vi "MM9.ProcCases.vi"(0 "i ref in":refnum<vi>, 1 "selector":string, 2 "Data":T1, 3 "call cluster":T3={"Object"="", "Selector"="", "CallType"=enum."synchronous", "Async Object"="", "Async Selector"="", "Data Descriptor"="", "Data"=[], "Error #"=0, "Expire"=0}, 5 "error in (no error)":errorcluster) -> (14 "i ref out":refnum<vi>, 17 "answer cluster":T3={"Object"="", "Selector"="", "CallType"=enum."synchronous", "Async Object"="", "Async Selector"="", "Data Descriptor"="", "Data"=[], "Error #"=0, "Expire"=0}, 19 "error out":errorcluster)   [LabVIEW 2014, in "MM9.lvlib"]
doc: "This method is called by a process from within the default case in the event loop. The methods of a class that are linked to events will be called from THIS method. Add your code here."
uses:
  MM9.lvlib
  CS_Core/CSSystem/CoreDefs/CoreDefs.call_type.ctl
  CS_Core/BaseProcess/BaseProcess.descriptor string definition.ctl
  CS_Core/CSSystem/CoreDefs/CoreDefs.rawDataType.ctl
  MM9.status.ctl
  CS_Core/CSSystem/CoreLib/CoreLib.byte array 2 string.vi
  CS_Core/CSSystem/CoreLib/CoreLib.string 2 byte array.vi
  CS_Core/BaseProcess/BaseProcess.lvlib
  CS_Core/CSSystem/CoreLib/CoreLib.lvlib
  CS_Core/CSSystem/CSSystemLib/CSSystemLib.lvlib
  CSlibraries-extern/DimLVEvent/LVDimInterface/LVDimInterface.lvlib
panel:
  in  "MMStatus":T2=enum."config"
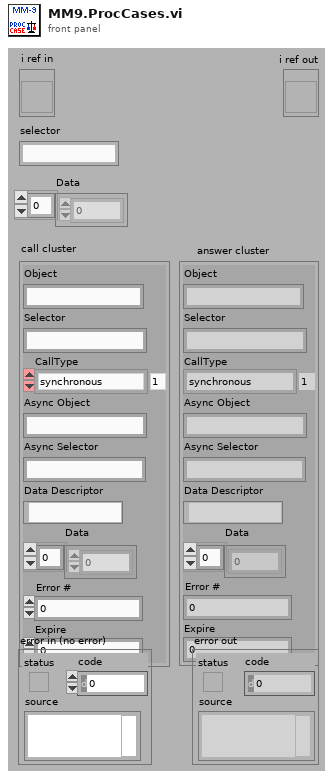
[diagram p1: front panel]
types:
  T1 = typedef "CoreDefs.rawDataType.ctl" = i8[]
  T2 = typedef "MM9.lvlib/MM9.status.ctl" = enum16{"loaded", "load_error", "config", "config_error", "init", "init_error", "data_reset", "data_reset_error", "running", "start_error", "run_error", "abort_requested", "aborted", "stop_requested", "stopped", "stop_error", "Connected", "NOTConnected"}
  T3 = typedef "CoreDefs.call_type.ctl" = cluster{"Object":string, "Selector":string, "CallType":enum16{"simple", "synchronous", "asynchronous"}, "Async Object":string, "Async Selector":string, "Data Descriptor":T4, "Data":T1, "Error #":i32, "Expire":u32}
  T4 = typedef "BaseProcess.lvlib/BaseProcess.descriptor string definition.ctl" = string
  T5 = typedef "MM9.lvlib/MM9.i attribute.ctl" = cluster{"UsedObjs":string[], "ActScanStep":i32[], "AbortRequest":bool, "StopRequest":bool, "# cycles":i32, "Connected":bool, "MMStatus":T2, "# data":i32, "DIMServices":cluster{"MM6StatusString":string, "MM6StatusID":i32, "discArchiver":string, "discArchiverID":i32, "eventBuilder":string, "eventBuilderID":i32, "GUIIDString":string, "GUIIDStringID":i32}, "dataFile":string, "PGRunning":T6, "ConfigData":T7, "ExtraDataSets":T22}
  T6 = typedef "PPG_ABC.lvlib/PPG_ABC.PG_Running.ctl" = i32
  T7 = typedef "LEBITDefs9.lvlib/LEBITDefs.ConfigData.ctl" = cluster{"GenConfig":T8, "Configs":T10[]}
  T8 = typedef "LEBITDefs9.lvlib/LEBITDefs.GenConfig.ctl" = cluster{"Mode":i32, "Logs":T9[]}
  T9 = typedef "LEBITDefs9.lvlib/LEBITDefs.Log.ctl" = cluster{"Name":string, "FctName":string, "Special":string}
  T10 = typedef "LEBITDefs9.lvlib/LEBITDefs.OneConfig.ctl" = cluster{"MCA":T11, "Timing":T12, "Scans":T15[], "FreqDevs":T16[], "CleanDev":T17, "NrCycles":i32, "Specials":T19[], "Delays":T20[], "DAC":T21}
  T11 = typedef "LEBITDefs9.lvlib/LEBITDefs.MCA.ctl" = cluster{"Name":string, "Address":string, "NrChannels":i32, "Gate":i32, "NrPipse":i32, "AcqDelay":i32}
  T12 = typedef "LEBITDefs9.lvlib/LEBITDefs.Timing.ctl" = cluster{"TimeTables":cluster{"TimeTable":T13}[], "Memories":T14[], "ScanX":string, "ScanY":string}
  T13 = typedef "LEBITDefs9.lvlib/LEBITDefs.Timetable.ctl" = dbl[]
  T14 = typedef "LEBITDefs9.lvlib/LEBITDefs.Memory.ctl" = cluster{"Device":string, "ExtTrig":bool, "TT2Use":i32, "PatternTable":string[]}
  T15 = typedef "LEBITDefs9.lvlib/LEBITDefs.ScanDev.ctl" = cluster{"Name":string, "FctName":string, "Values":dbl[], "NrScanVals":i32, "Special":string}
  T16 = typedef "LEBITDefs9.lvlib/LEBITDefs.FreqDev.ctl" = cluster{"Name":string, "Amp":dbl, "CenterFreq":dbl, "Time":dbl}
  T17 = typedef "LEBITDefs9.lvlib/LEBITDefs.CleanDev.ctl" = cluster{"Name":string, "CleanData":T18[]}
  T18 = typedef "LEBITDefs9.lvlib/LEBITDefs.CleanDataType.ctl" = cluster{"Amp":dbl, "Center":dbl, "Plus":dbl, "Minus":dbl, "Time":dbl}
  T19 = typedef "LEBITDefs9.lvlib/LEBITDefs.Special.ctl" = cluster{"Name":string, "FctName":string, "VerySpecial":string, "Data":dbl}
  T20 = typedef "LEBITDefs9.lvlib/LEBITDefs.Delay.ctl" = cluster{"Name":string, "Delay":dbl}
  T21 = typedef "LEBITDefs9.lvlib/LEBITDefs.DAC.ctl" = cluster{"Name":string, "Step1":i32, "Step2":i32}
  T22 = typedef "LEBITDefs9.lvlib/LEBITDefs.ExtraData.ctl" = cluster{"Ions":cluster{"ExcitIonMass":string, "ExcitIonCharge":i32, "CleanIons":cluster{"CleanIonMass":string, "CleanIonCharge":i32}[]}, "TimingDescription":cluster{"TimeTableDescription":cluster{"Times":string[]}[], "PatternTableDescription":cluster{"Pattern":string[]}[]}, "ScanUnits":string[]}[]
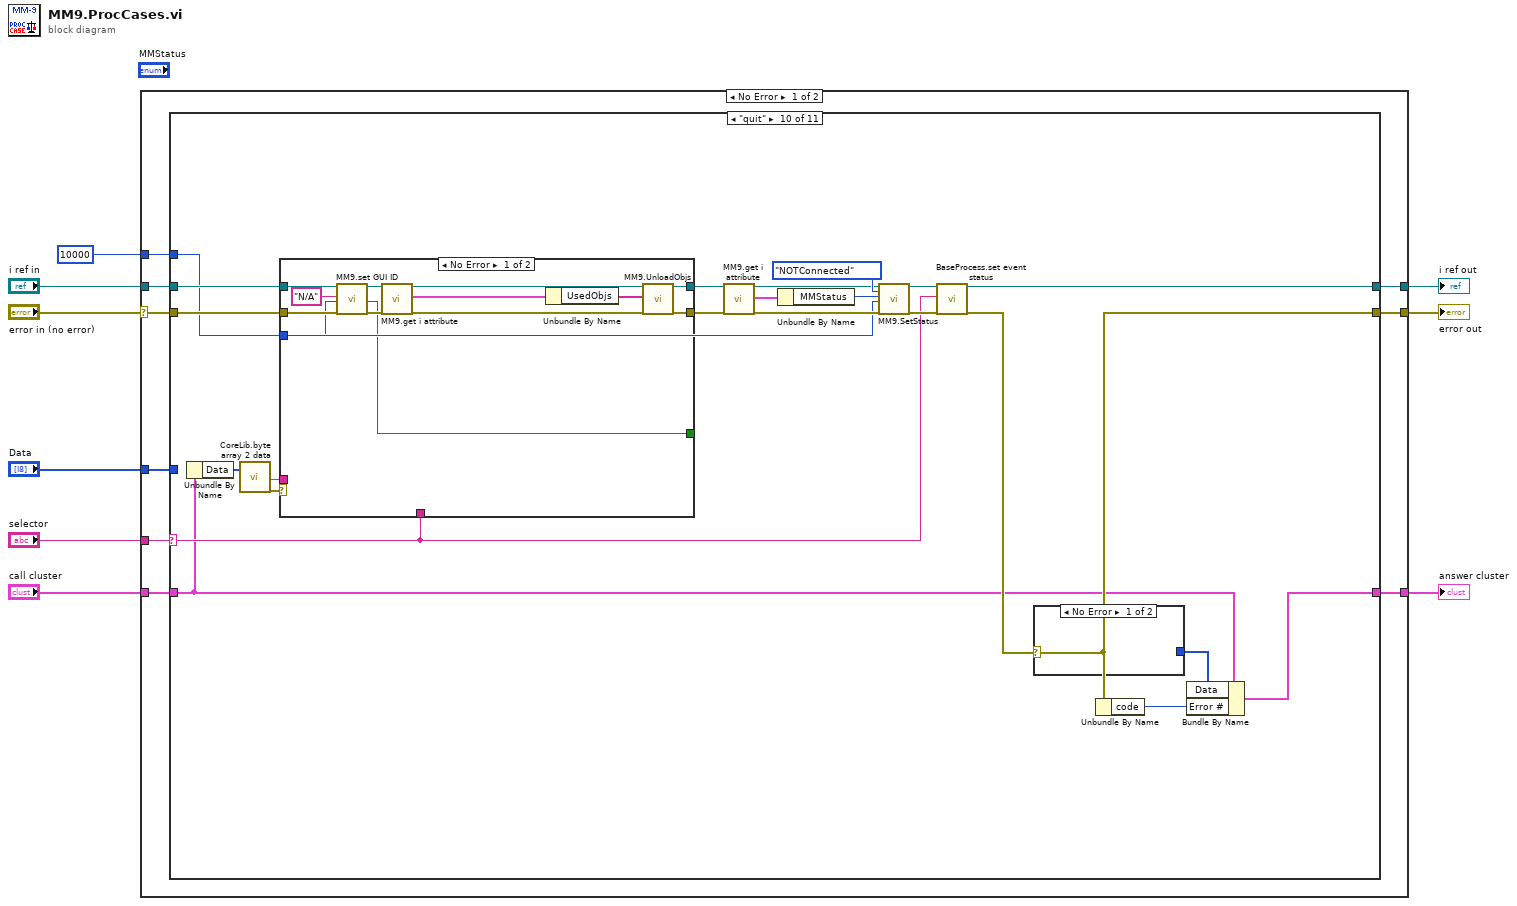
[diagram p0: block diagram]
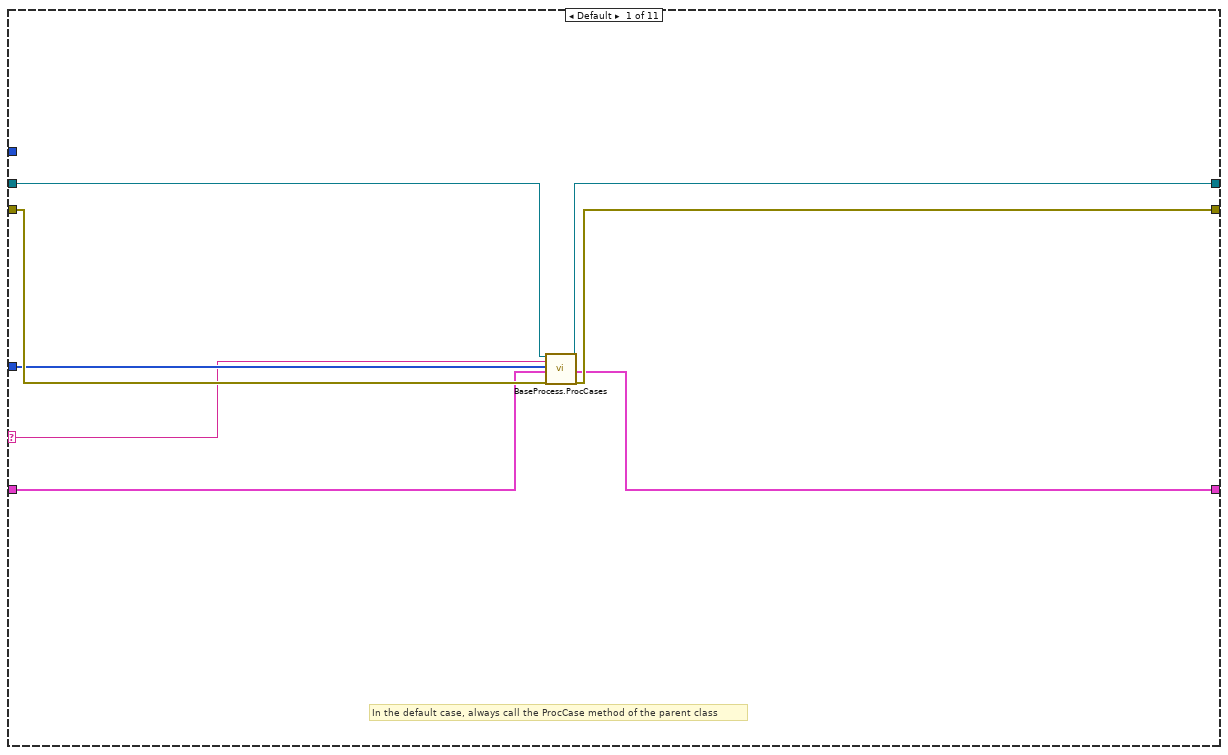
[diagram p2: hidden frame]
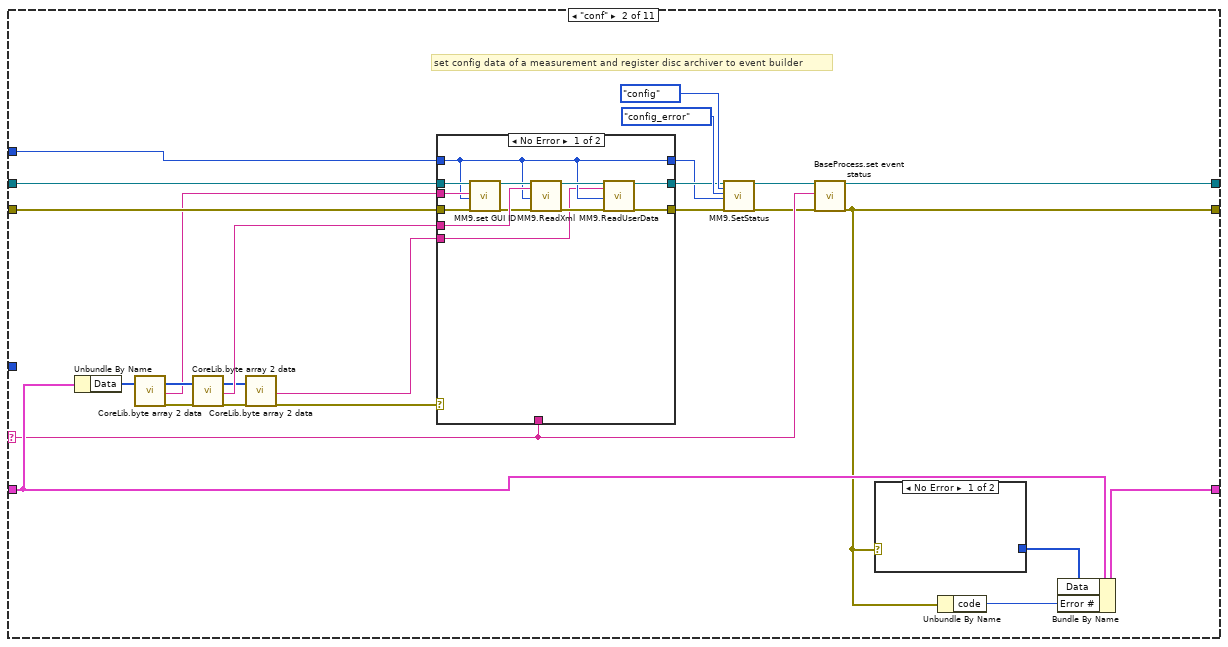
[diagram p3: hidden frame]
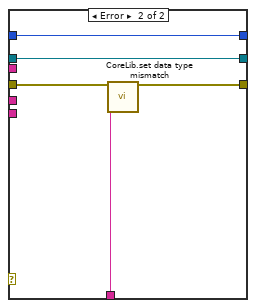
[diagram p4: hidden frame]
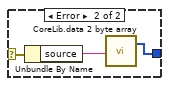
[diagram p5: hidden frame]
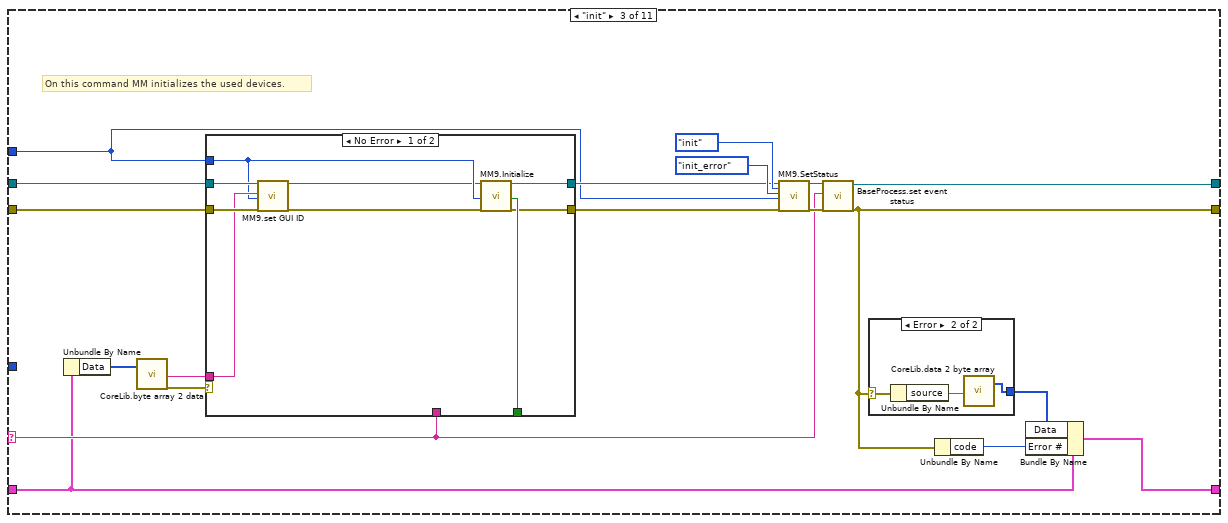
[diagram p6: hidden frame]
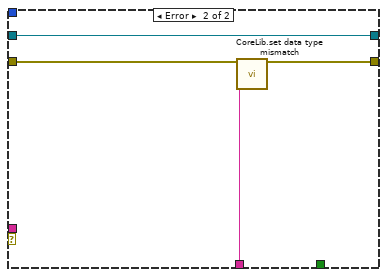
[diagram p7: hidden frame]
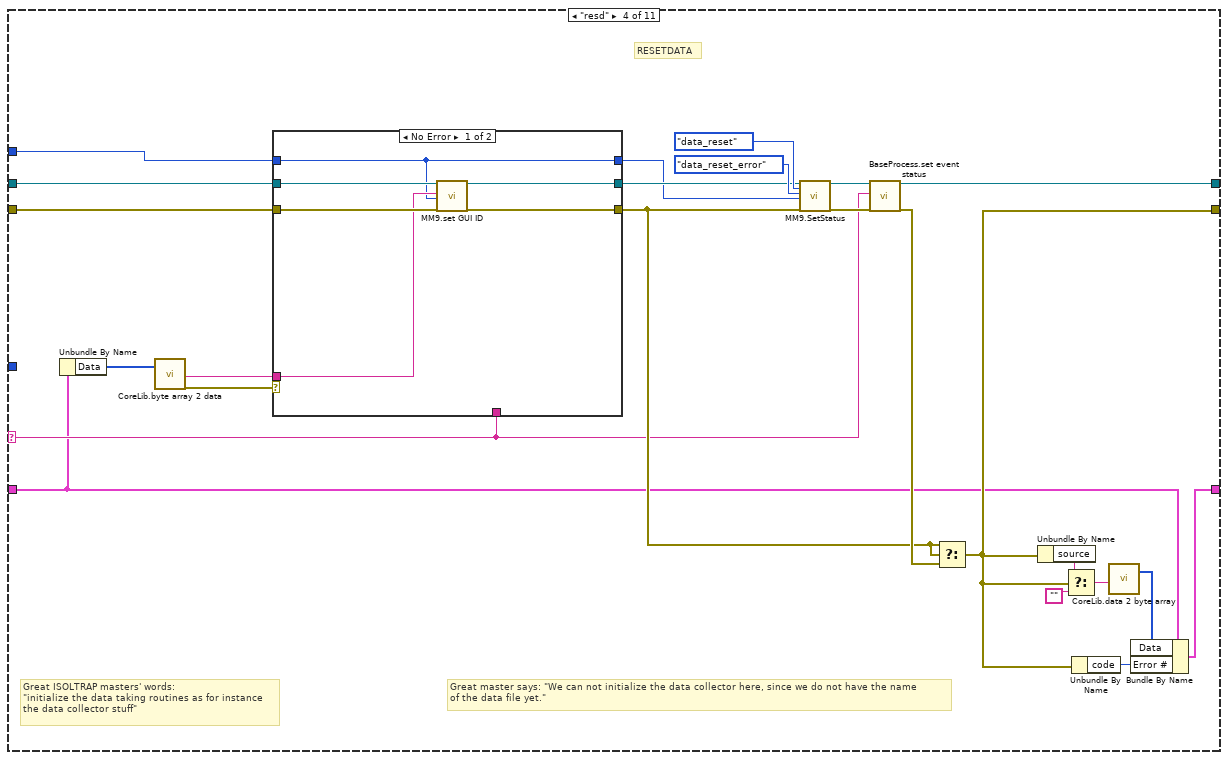
[diagram p9: hidden frame]
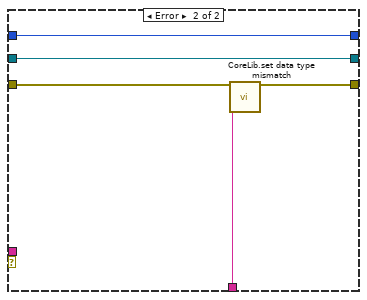
[diagram p10: hidden frame]
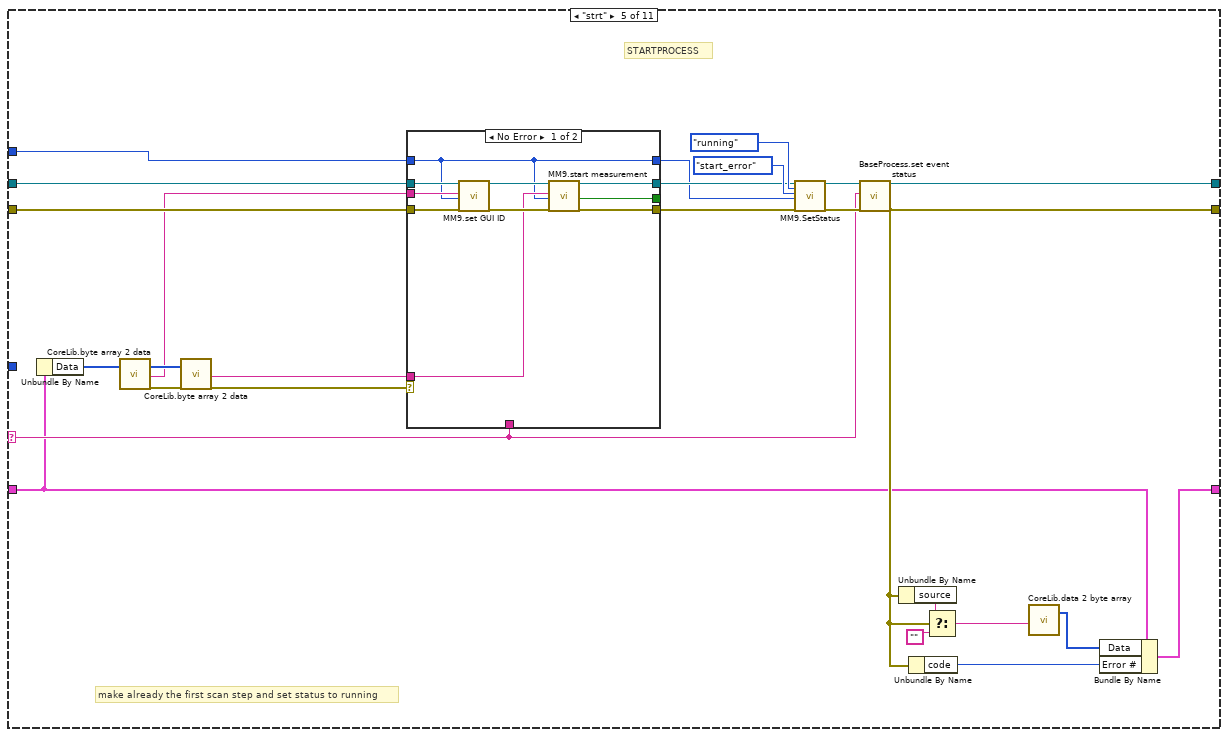
[diagram p11: hidden frame]
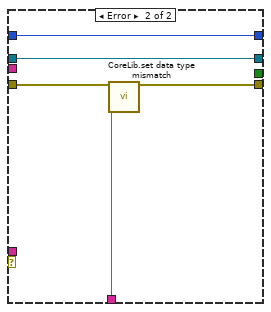
[diagram p12: hidden frame]
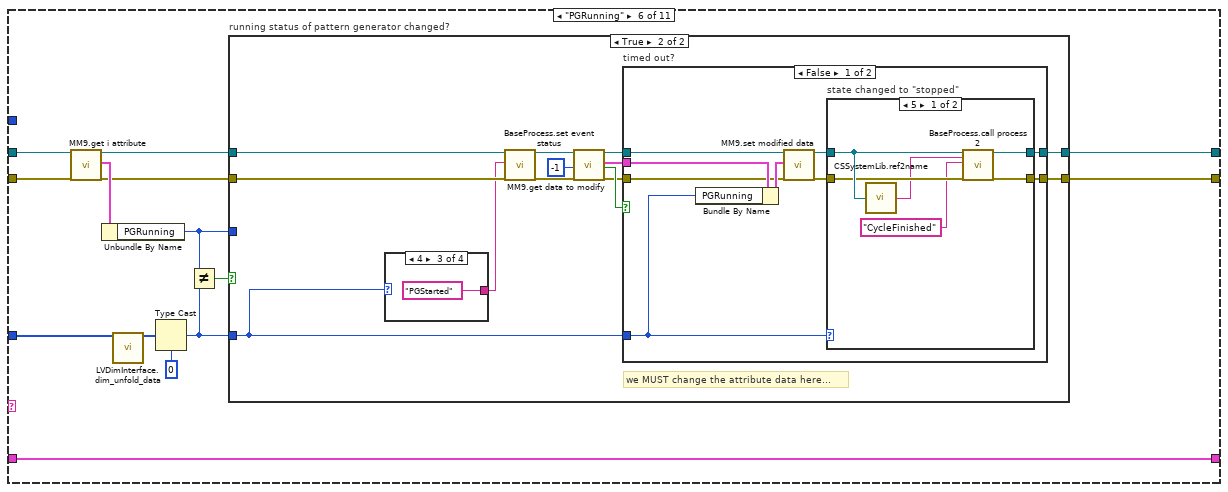
[diagram p13: hidden frame]
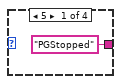
[diagram p15: hidden frame]
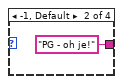
[diagram p16: hidden frame]
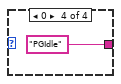
[diagram p17: hidden frame]
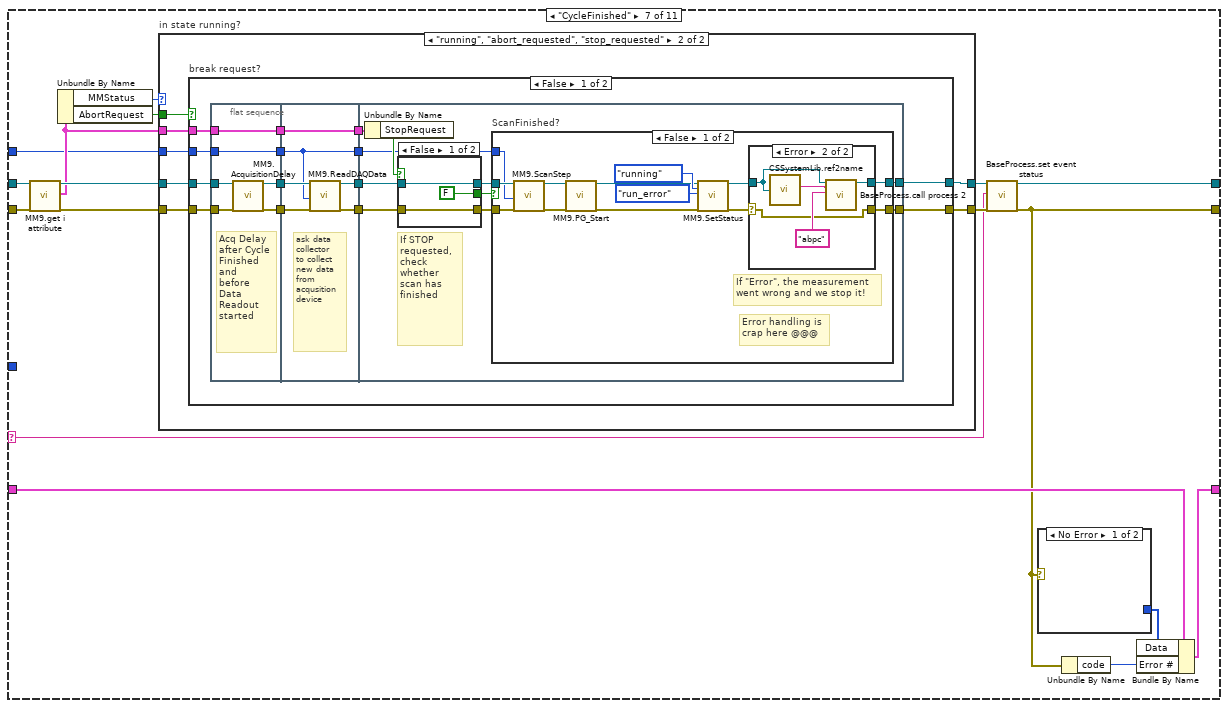
[diagram p20: hidden frame]
diagram:
  n1 = case shown="No Error" "error in (no error)" {
    selector: "error in (no error)" -> [w10 w537]
    tunnel: [w18 w538] -> w9
    tunnel: "call cluster" -> [w17 w538]
    tunnel: [w16 w539] -> w7
    tunnel: [w15 w537] -> w6
    tunnel: "i ref in" -> [w14 w539]
    tunnel: "selector" -> [w13 _]
    tunnel: 10000 ("ms timeout (100)") -> [w12 _]
    tunnel: "Data" -> [w11 _]
    frame No Error {
      n2 = case shown="\"quit\"" w13 {
        selector: w13 -> [w20 w46 w75 w113 w148 _ w237 w348 w408 w460 w502]
        tunnel: w11 -> [w21 _ _ _ _ w197 _ _ _ _ _]
        tunnel: [w26 w41 w81 w129 w168 w186 w241 w364 w423 w479 w522] -> w16
        tunnel: w17 -> [w22 w50 w73 w109 w143 w187 w248 w347 w407 w459 w501]
        tunnel: [w23 w49 w91 w130 w166 w187 w247 w365 w424 w477 w520] -> w18
        tunnel: w10 -> [w25 w32 w78 w114 w153 w193 w251 w368 w427 w464 w507]
        tunnel: [w24 w48 w90 w125 w163 w188 w240 w363 w422 w478 w521] -> w15
        tunnel: w12 -> [_ w36 w80 w112 w151 _ w238 w352 w412 w463 w504]
        tunnel: w14 -> [w19 w33 w79 w116 w155 w194 w252 w369 w428 w465 w510]
        frame Default {
          # "In the default case, always call the ProcCase method of the parent class"
          n3 = call "BaseProcess.ProcCases.vi"("i ref in"=w19, "selector"=w20, "Data"=w21, "call cluster"=w22, "error in (no error)"=w25) -> ("i ref out"=w26:refnum<vi>, "answer cluster"=w23:T3, "error out"=w24:errorcluster)  [unwired: 12 in]
        }
        frame "conf" {
          # "set config data of a measurement and register disc archiver to event builder"
          n4 = Unbundle By Name(w50) -> ("Data"=w47:T1)
          n5 = call-poly "CoreLib.byte array 2 data.vi"("byteArray"=w47) -> ("byteArray out"=w40:T1, "string"=w31:string, "error out"=w39:errorcluster)  [unwired: 16 in]
          n6 = call-poly "CoreLib.byte array 2 data.vi"("byteArray"=w40, "error in (no error)"=w39) -> ("byteArray out"=w29:T1, "string"=w34:string, "error out"=w30:errorcluster)  [unwired: 15 in]
          n7 = call-poly "CoreLib.byte array 2 data.vi"("byteArray"=w29, "error in (no error)"=w30) -> ("string"=w28:string, "error out"=w27:errorcluster)  [unwired: 15 in, 1 out]
          n8 = case shown="No Error" w27 {
            tunnel: [w55 w68] -> w42
            tunnel: w46 -> [_ w69]
            tunnel: w32 -> [w62 w67]
            tunnel: w33 -> [w63 w66]
            tunnel: [w56 w66] -> w37
            tunnel: w36 -> [w54 w65]
            tunnel: [w54 w65] -> w35
            tunnel: w34 -> [w64 _]
            tunnel: w31 -> [w61 _]
            tunnel: w28 -> [w53 _]
            frame No Error {
              n9 = call "MM9.set GUI ID.vi"("i ref in"=w63, "GUIDString"=w61, "ms timeout (10000)"=w54, "error in (no error)"=w62) -> ("i ref out"=w60:refnum<vi>, "error out"=w59:errorcluster)  [unwired: 13 in, 1 out]
              n10 = call "MM9.ReadXml.vi"("i ref in"=w60, "Data"=w64, "timeout ms"=w54, "error in (no error)"=w59) -> ("i ref out"=w58:refnum<vi>, "error out"=w57:errorcluster)  [unwired: 13 in, 1 out]
              n11 = call "MM9.ReadUserData.vi"("i ref in"=w58, "Data"=w53, "timeout ms"=w54, "error in (no error)"=w57) -> ("i ref out"=w56:refnum<vi>, "error out"=w55:errorcluster)  [unwired: 13 in, 1 out]
            }
            frame Error {
              n12 = call "CoreLib.set data type mismatch.vi"("error in (no error)"=w67, "error source"=w69) -> ("error out"=w68:errorcluster)  [unwired: 17 in]
            }
          }
          n13 = call "MM9.SetStatus.vi"("i ref in"=w37, "MMStatusSuccess"=MM9.status."config" ("MMStatus"), "MMStatusFail"=MM9.status."config_error" ("MMStatus"), "ms timeout (10000)"=w35, "error in (no error)"=w42) -> ("i ref out"=w44:refnum<vi>, "error out"=w43:errorcluster)  [unwired: 11 in, 2 out]
          n14 = call "BaseProcess.set event status.vi"("i ref in"=w44, "EventStatus"=w46, "error in (no error)"=w43) -> ("i ref out"=w41:refnum<vi>, "error out"=w48:errorcluster)  [unwired: 14 in, 1 out]
          n15 = case shown="No Error" w48 {
            selector: w48 -> [_ w72]
            tunnel: [_ w71] -> w52
            frame No Error {
            }
            frame Error {
              n16 = Unbundle By Name(w72) -> ("source"=w70:string)
              n17 = call-poly "CoreLib.data 2 byte array.vi"("string"=w70) -> ("byteArray out"=w71:T1)  [unwired: 18 in]
            }
          }
          n18 = Unbundle By Name(w48) -> ("code"=w51:i32)
          n19 = Bundle By Name(cluster=w50, "Data"=w52, "Error #"=w51) -> (w49:T3)
        }
        frame "init" {
          # "On this command MM initializes the used devices."
          n20 = Unbundle By Name(w73) -> ("Data"=w74:T1)
          n21 = call-poly "CoreLib.byte array 2 data.vi"("byteArray"=w74) -> ("string"=w76:string, "error out"=w77:errorcluster)  [unwired: 16 in, 1 out]
          n22 = case shown="No Error" w77 {
            tunnel: [w100 _] -> _
            tunnel: [w99 w103] -> w85
            tunnel: [w98 w102] -> w84
            tunnel: w80 -> [w94 _]
            tunnel: w79 -> [w97 w102]
            tunnel: w78 -> [w96 w104]
            tunnel: w76 -> [w95 _]
            tunnel: w75 -> [_ w101]
            frame No Error {
              n23 = call "MM9.set GUI ID.vi"("i ref in"=w97, "GUIDString"=w95, "ms timeout (10000)"=w94, "error in (no error)"=w96) -> ("i ref out"=w93:refnum<vi>, "error out"=w92:errorcluster)  [unwired: 13 in, 1 out]
              n24 = call "MM9.Initialize.vi"("i ref in"=w93, "ms timeout (10000)"=w94, "error in (no error)"=w92) -> ("i ref out"=w98:refnum<vi>, "timed out"=w100:bool, "error out"=w99:errorcluster)  [unwired: 14 in]
            }
            frame Error {
              n25 = call "CoreLib.set data type mismatch.vi"("error in (no error)"=w104, "error source"=w101) -> ("error out"=w103:errorcluster)  [unwired: 17 in]
            }
          }
          n26 = call "MM9.SetStatus.vi"("i ref in"=w84, "MMStatusSuccess"=MM9.status."init" ("MMStatus"), "MMStatusFail"=MM9.status."init_error" ("MMStatus"), "ms timeout (10000)"=w80, "error in (no error)"=w85) -> ("i ref out"=w83:refnum<vi>, "error out"=w82:errorcluster)  [unwired: 11 in, 2 out]
          n27 = call "BaseProcess.set event status.vi"("i ref in"=w83, "EventStatus"=w75, "error in (no error)"=w82) -> ("i ref out"=w81:refnum<vi>, "error out"=w90:errorcluster)  [unwired: 14 in, 1 out]
          n28 = case shown="Error" w90 {
            selector: w90 -> [_ w107]
            tunnel: [_ w105] -> w89
            frame No Error {
            }
            frame Error {
              n29 = Unbundle By Name(w107) -> ("source"=w106:string)
              n30 = call-poly "CoreLib.data 2 byte array.vi"("string"=w106) -> ("byteArray out"=w105:T1)  [unwired: 18 in]
            }
          }
          n31 = Unbundle By Name(w90) -> ("code"=w88:i32)
          n32 = Bundle By Name(cluster=w73, "Data"=w89, "Error #"=w88) -> (w91:T3)
        }
        frame "resd" {
          # "Great master says: \"We can not initialize the data collector here, since we do not have the name\nof the data file yet.\""
          # "RESETDATA"
          # "Great ISOLTRAP masters' words:\n\"initialize the data taking routines as for instance\nthe data collector stuff\""
          n33 = Unbundle By Name(w109) -> ("Data"=w108:T1)
          n34 = call-poly "CoreLib.byte array 2 data.vi"("byteArray"=w108) -> ("string"=w110:string, "error out"=w115:errorcluster)  [unwired: 16 in, 1 out]
          n35 = case shown="No Error" w115 {
            tunnel: [w133 w139] -> w118
            tunnel: [w132 w141] -> w117
            tunnel: w116 -> [w137 w139]
            tunnel: w114 -> [w136 w142]
            tunnel: w113 -> [_ w140]
            tunnel: w112 -> [w134 w138]
            tunnel: [w134 w138] -> w111
            tunnel: w110 -> [w135 _]
            frame No Error {
              n36 = call "MM9.set GUI ID.vi"("i ref in"=w137, "GUIDString"=w135, "ms timeout (10000)"=w134, "error in (no error)"=w136) -> ("i ref out"=w133:refnum<vi>, "error out"=w132:errorcluster)  [unwired: 13 in, 1 out]
            }
            frame Error {
              n37 = call "CoreLib.set data type mismatch.vi"("error in (no error)"=w142, "error source"=w140) -> ("error out"=w141:errorcluster)  [unwired: 17 in]
            }
          }
          n38 = call "MM9.SetStatus.vi"("i ref in"=w118, "MMStatusSuccess"=MM9.status."data_reset" ("MMStatus"), "MMStatusFail"=MM9.status."data_reset_error" ("MMStatus"), "ms timeout (10000)"=w111, "error in (no error)"=w117) -> ("i ref out"=w122:refnum<vi>, "error out"=w121:errorcluster)  [unwired: 11 in, 2 out]
          n39 = call "BaseProcess.set event status.vi"("i ref in"=w122, "EventStatus"=w113, "error in (no error)"=w121) -> ("i ref out"=w129:refnum<vi>, "error out"=w128:errorcluster)  [unwired: 14 in, 1 out]
          n40 = Select(t=w117, s=w117, f=w128) -> (s? t:f=w125:errorcluster)
          n41 = Unbundle By Name(w125) -> ("source"=w127:string)
          n42 = Select(t=w127, s=w125, f="") -> (s? t:f=w120:string)
          n43 = Unbundle By Name(w125) -> ("code"=w131:i32)
          n44 = call-poly "CoreLib.data 2 byte array.vi"("string"=w120) -> ("byteArray out"=w119:T1)  [unwired: 18 in]
          n45 = Bundle By Name(cluster=w109, "Data"=w119, "Error #"=w131) -> (w130:T3)
        }
        frame "strt" {
          # "STARTPROCESS"
          # "make already the first scan step and set status to running"
          n46 = Unbundle By Name(w143) -> ("Data"=w144:T1)
          n47 = call-poly "CoreLib.byte array 2 data.vi"("byteArray"=w144) -> ("byteArray out"=w156:T1, "string"=w147:string, "error out"=w145:errorcluster)  [unwired: 16 in]
          n48 = call-poly "CoreLib.byte array 2 data.vi"("byteArray"=w156, "error in (no error)"=w145) -> ("string"=w146:string, "error out"=w150:errorcluster)  [unwired: 15 in, 1 out]
          n49 = case shown="No Error" w150 {
            tunnel: w155 -> [w178 w183]
            tunnel: [w176 w183] -> w154
            tunnel: w153 -> [w175 w182]
            tunnel: [w173 w181] -> w152
            tunnel: w151 -> [w170 w180]
            tunnel: [w170 w180] -> w149
            tunnel: w148 -> [_ w179]
            tunnel: w147 -> [w172 _]
            tunnel: w146 -> [w171 _]
            tunnel: [w169 _] -> _
            frame No Error {
              n50 = call "MM9.set GUI ID.vi"("i ref in"=w178, "GUIDString"=w172, "ms timeout (10000)"=w170, "error in (no error)"=w175) -> ("i ref out"=w177:refnum<vi>, "error out"=w174:errorcluster)  [unwired: 13 in, 1 out]
              n51 = call "MM9.start measurement.vi"("i ref in"=w177, "dataFileName"=w171, "ms timeout (10000)"=w170, "error in (no error)"=w174) -> ("i ref out"=w176:refnum<vi>, "timed out"=w169:bool, "error out"=w173:errorcluster)  [unwired: 13 in]
            }
            frame Error {
              n52 = call "CoreLib.set data type mismatch.vi"("error in (no error)"=w182, "error source"=w179) -> ("error out"=w181:errorcluster)  [unwired: 17 in]
            }
          }
          n53 = call "MM9.SetStatus.vi"("i ref in"=w154, "MMStatusSuccess"=MM9.status."running" ("MMStatus"), "MMStatusFail"=MM9.status."start_error" ("MMStatus"), "ms timeout (10000)"=w149, "error in (no error)"=w152) -> ("i ref out"=w159:refnum<vi>, "error out"=w160:errorcluster)  [unwired: 11 in, 2 out]
          n54 = call "BaseProcess.set event status.vi"("i ref in"=w159, "EventStatus"=w148, "error in (no error)"=w160) -> ("i ref out"=w168:refnum<vi>, "error out"=w163:errorcluster)  [unwired: 14 in, 1 out]
          n55 = Unbundle By Name(w163) -> ("source"=w165:string)
          n56 = Unbundle By Name(w163) -> ("code"=w167:i32)
          n57 = Select(t=w165, s=w163, f="") -> (s? t:f=w157:string)
          n58 = call-poly "CoreLib.data 2 byte array.vi"("string"=w157) -> ("byteArray out"=w158:T1)  [unwired: 18 in]
          n59 = Bundle By Name(cluster=w143, "Data"=w158, "Error #"=w167) -> (w166:T3)
        }
        frame "PGRunning" {
          n60 = call "MM9.get i attribute.vi"("i ref in"=w194, "error in (no error)"=w193) -> ("i ref out"=w190:refnum<vi>, "i attribute"=w192:T5, "error out"=w189:errorcluster)  [unwired: 15 in]
          n61 = Unbundle By Name(w192) -> ("PGRunning"=w185:T6)
          n62 = call "LVDimInterface.dim_unfold_data.vi"("rawData"=w197) -> ("data"=w195:i8[])  [unwired: 15 in, 3 out]
          n63 = Type Cast(type=0, x=w195) -> (*(type *) &x=w184:i32)
          n64 = Not Equal?(x=w185, y=w184) -> (x != y?=w191:bool)
          n65 = case "running status of pattern generator changed?" shown="True" w191 {
            tunnel: w190 -> [w199 w205]
            tunnel: w189 -> [w198 w204]
            tunnel: [w198 w206] -> w188
            tunnel: [w199 w207] -> w186
            tunnel: w185 -> [_ _]
            tunnel: w184 -> [_ w201]
            frame False {
            }
            frame True {
              # "we MUST change the attribute data here..."
              n66 = case shown="4" w201 {
                tunnel: ["PGStopped" "PG - oh je!" "PGStarted" "PGIdle"] -> w200
                frame 5 {
                }
                frame -1, Default {
                }
                frame 4 {
                }
                frame 0 {
                }
              }
              n67 = call "BaseProcess.set event status.vi"("i ref in"=w205, "EventStatus"=w200, "error in (no error)"=w204) -> ("i ref out"=w203:refnum<vi>, "error out"=w202:errorcluster)  [unwired: 14 in, 1 out]
              n68 = call "MM9.get data to modify.vi"("i ref in"=w203, "ms timeout (10000)"=-1, "error in (no error)"=w202) -> ("i ref out"=w209:refnum<vi>, "i attribute"=w208:T5, "timed out"=w212:bool, "error out"=w210:errorcluster)  [unwired: 13 in]
              n69 = case "timed out?" shown="False" w212 {
                tunnel: w210 -> [w219 w234]
                tunnel: w209 -> [w225 w235]
                tunnel: [w217 w235] -> w207
                tunnel: [w218 w234] -> w206
                tunnel: w208 -> [w224 _]
                tunnel: w201 -> [w222 _]
                frame False {
                  n70 = Bundle By Name(cluster=w224, "PGRunning"=w222) -> (w223:T5)
                  n71 = call "MM9.set modified data.vi"("i ref in"=w225, "i attribute"=w223, "error in (no error)"=w219) -> ("i ref out"=w221:refnum<vi>, "error out"=w220:errorcluster)  [unwired: 15 in]
                  n72 = case "state changed to \"stopped\"" shown="5" w222 {
                    tunnel: w221 -> [w231 w233]
                    tunnel: w220 -> [w230 w232]
                    tunnel: [w229 w232] -> w218
                    tunnel: [w228 w233] -> w217
                    frame 5 {
                      n73 = call "CSSystemLib.ref2name.vi"("obj refnum"=w231) -> ("name"=w227:string)
                      n74 = call "BaseProcess.call process 2.vi"("i ref in"=w231, "Object"=w227, "Selector"="CycleFinished", "error in (no error)"=w230) -> ("i ref out"=w228:refnum<vi>, "error out"=w229:errorcluster)  [unwired: 14 in]
                    }
                    frame Default {
                    }
                  }
                }
                frame True {
                }
              }
            }
          }
        }
        frame "CycleFinished" {
          n75 = call "MM9.get i attribute.vi"("i ref in"=w252, "error in (no error)"=w251) -> ("i ref out"=w246:refnum<vi>, "i attribute"=w243:T5, "error out"=w245:errorcluster)  [unwired: 15 in]
          n76 = Unbundle By Name(w243) -> ("MMStatus"=w236:T2, "AbortRequest"=w244:bool)
          n77 = case "in state running?" shown="\"running\", \"abort_requested\", \"stop_requested\"" w236 {
            tunnel: w246 -> [w254 w261]
            tunnel: w245 -> [w253 w260]
            tunnel: w244 -> [_ w259]
            tunnel: w243 -> [_ w258]
            tunnel: [w254 w257] -> w242
            tunnel: [w253 w256] -> w239
            tunnel: w238 -> [_ w255]
            frame Default {
            }
            frame "running", "abort_requested", "stop_requested" {
              n78 = case "break request?" shown="False" w259 {
                tunnel: [w272 w340] -> w257
                tunnel: w261 -> [w275 w337]
                tunnel: w260 -> [w274 w336]
                tunnel: [w271 w339] -> w256
                tunnel: w258 -> [w273 _]
                tunnel: w255 -> [w270 w338]
                frame False {
                  n79 = flat-sequence {
                    tunnel: w275 -> [w279]
                    tunnel: w274 -> [w278]
                    tunnel: w273 -> [w281]
                    tunnel: [w281] -> w268
                    tunnel: w270 -> [w280]
                    tunnel: [w280] -> w266
                    tunnel: [w277] -> w263
                    tunnel: [w276] -> w262
                    tunnel: [w285] -> w269
                    tunnel: w268 -> [w287]
                    tunnel: [w287] -> w267
                    tunnel: w266 -> [w282]
                    tunnel: [w282] -> w265
                    tunnel: [w284] -> w264
                    tunnel: w263 -> [w286]
                    tunnel: w262 -> [w283]
                    tunnel: w269 -> [w296]
                    tunnel: w267 -> [w297]
                    tunnel: [w290] -> w272
                    tunnel: [w289] -> w271
                    tunnel: w265 -> [w291]
                    tunnel: w264 -> [w288]
                    frame #0 {
                      # "Acq Delay\nafter Cycle\nFinished\nand\nbefore\nData\nReadout\nstarted"
                      n80 = call "MM9.AcquisitionDelay.vi"("i ref in"=w279, "error in (no error)"=w278) -> ("i ref out"=w277:refnum<vi>, "error out"=w276:errorcluster)  [unwired: 16 in]
                    }
                    frame #1 {
                      # "ask data collector\nto collect new data\nfrom acqusition device"
                      n81 = call "MM9.ReadDAQData.vi"("i ref in"=w286, "ms timeout (10000)"=w282, "error in (no error)"=w283) -> ("i ref out"=w285:refnum<vi>, "error out"=w284:errorcluster)  [unwired: 14 in, 1 out]
                    }
                    frame #2 {
                      # "If STOP requested, check whether scan has finished"
                      n82 = Unbundle By Name(w297) -> ("StopRequest"=w295:bool)
                      n83 = case shown="False" w295 {
                        tunnel: w296 -> [w328 w333]
                        tunnel: [FALSE ("ScanFini") w332] -> w294
                        tunnel: [w328 w331] -> w293
                        tunnel: [w327 w330] -> w292
                        tunnel: w288 -> [w327 w329]
                        frame False {
                        }
                        frame True {
                          n84 = call "MM9.IsScanFinished.vi"("i ref in"=w333, "error in (no error)"=w329) -> ("i ref out"=w331:refnum<vi>, "ScanFini"=w332:bool, "error out"=w330:errorcluster)  [unwired: 15 in]
                        }
                      }
                      n85 = case "ScanFinished?" shown="False" w294 {
                        tunnel: [w310 w325] -> w290
                        tunnel: [w309 w324] -> w289
                        tunnel: w293 -> [w308 w319]
                        tunnel: w292 -> [w307 w318]
                        tunnel: w291 -> [w298 _]
                        frame False {
                          # "Error handling is\ncrap here @@@"
                          # "If \"Error\", the measurement\nwent wrong and we stop it!"
                          n86 = call "MM9.ScanStep.vi"("i ref in"=w308, "ms timeout (10000)"=w298, "error in (no error)"=w307) -> ("i ref out"=w306:refnum<vi>, "error out"=w305:errorcluster)  [unwired: 14 in, 1 out]
                          n87 = call "MM9.PG_Start.vi"("i ref in"=w306, "error in (no error)"=w305) -> ("i ref out"=w302:refnum<vi>, "error out"=w301:errorcluster)  [unwired: 16 in]
                          n88 = call "MM9.SetStatus.vi"("i ref in"=w302, "MMStatusSuccess"=MM9.status."running", "MMStatusFail"=MM9.status."run_error", "error in (no error)"=w301) -> ("i ref out"=w299:refnum<vi>, "error out"=w300:errorcluster)  [unwired: 12 in, 2 out]
                          n89 = case shown="Error" w300 {
                            selector: w300 -> [w312 w313]
                            tunnel: [w311 w317] -> w310
                            tunnel: w299 -> [w311 w314]
                            tunnel: [w312 w313] -> w309
                            frame No Error {
                            }
                            frame Error {
                              n90 = call "CSSystemLib.ref2name.vi"("obj refnum"=w314) -> ("name"=w316:string)
                              n91 = call "BaseProcess.call process 2.vi"("i ref in"=w314, "Object"=w316, "Selector"="abpc") -> ("i ref out"=w317:refnum<vi>)  [unwired: 15 in, 1 out]
                            }
                          }
                        }
                        frame True {
                          # "stop cycle controller...\n@@@@@@"
                          # "scan finished"
                          n92 = call "MM9.PG_Stop.vi"("i ref in"=w319, "error in (no error)"=w318) -> ("i ref out"=w322:refnum<vi>, "error out"=w323:errorcluster)  [unwired: 16 in]
                          n93 = call "MM9.SetStatus.vi"("i ref in"=w322, "MMStatusSuccess"=MM9.status."stopped" ("MMStatus"), "MMStatusFail"=MM9.status."stop_error" ("MMStatus"), "error in (no error)"=w323) -> ("i ref out"=w325:refnum<vi>, "error out"=w324:errorcluster)  [unwired: 12 in, 2 out]
                        }
                      }
                    }
                  }
                }
                frame True {
                  # "stop cyclecontroller..."
                  n94 = call "MM9.PG_Stop.vi"("i ref in"=w337, "error in (no error)"=w336) -> ("i ref out"=w334:refnum<vi>, "error out"=w335:errorcluster)  [unwired: 16 in]
                  n95 = call "MM9.SetStatus.vi"("i ref in"=w334, "MMStatusSuccess"=MM9.status."aborted" ("MMStatus"), "MMStatusFail"=MM9.status."stop_error" ("MMStatus"), "ms timeout (10000)"=w338, "error in (no error)"=w335) -> ("i ref out"=w340:refnum<vi>, "error out"=w339:errorcluster)  [unwired: 11 in, 2 out]
                }
              }
            }
          }
          n96 = call "BaseProcess.set event status.vi"("i ref in"=w242, "EventStatus"=w237, "error in (no error)"=w239) -> ("i ref out"=w241:refnum<vi>, "error out"=w240:errorcluster)  [unwired: 14 in, 1 out]
          n97 = case shown="No Error" w240 {
            selector: w240 -> [_ w345]
            tunnel: [_ w343] -> w250
            frame No Error {
            }
            frame Error {
              n98 = Unbundle By Name(w345) -> ("source"=w344:string)
              n99 = call-poly "CoreLib.data 2 byte array.vi"("string"=w344) -> ("byteArray out"=w343:T1)  [unwired: 18 in]
            }
          }
          n100 = Unbundle By Name(w240) -> ("code"=w249:i32)
          n101 = Bundle By Name(cluster=w248, "Data"=w250, "Error #"=w249) -> (w247:T3)
        }
        frame "abpc" {
          # "\"BREAKPROCESS\""
          # "Don't set the status\nhere. We want to\nkeep the status the\nhas occured before\nbreak was requested"
          n102 = Unbundle By Name(w347) -> ("Data"=w346:T1)
          n103 = call-poly "CoreLib.byte array 2 data.vi"("byteArray"=w346) -> ("string"=w349:string, "error out"=w350:errorcluster)  [unwired: 16 in, 1 out]
          n104 = case shown="No Error" w350 {
            tunnel: w369 -> [w375 w391]
            tunnel: w368 -> [w372 w394]
            tunnel: [w379 _] -> _
            tunnel: [w377 w391] -> w360
            tunnel: [w376 w393] -> w359
            tunnel: w352 -> [w370 w395]
            tunnel: [w370 w395] -> w351
            tunnel: w349 -> [w371 _]
            tunnel: w348 -> [_ w392]
            frame No Error {
              n105 = call "MM9.set GUI ID.vi"("i ref in"=w375, "GUIDString"=w371, "ms timeout (10000)"=w370, "error in (no error)"=w372) -> ("i ref out"=w373:refnum<vi>, "error out"=w374:errorcluster)  [unwired: 13 in, 1 out]
              n106 = call "MM9.get data to modify.vi"("i ref in"=w373, "ms timeout (10000)"=w370, "error in (no error)"=w374) -> ("i ref out"=w381:refnum<vi>, "i attribute"=w378:T5, "timed out"=w379:bool, "error out"=w380:errorcluster)  [unwired: 13 in]
              n107 = case "timed out?" shown="False" w379 {
                tunnel: w381 -> [w387 w390]
                tunnel: [w388 w390] -> w377
                tunnel: w380 -> [w386 w389]
                tunnel: [w385 w389] -> w376
                tunnel: w378 -> [w384 _]
                frame False {
                  n108 = Bundle By Name(cluster=w384, "AbortRequest"=TRUE ("BreakRequest")) -> (w383:T5)
                  n109 = call "MM9.set modified data.vi"("i ref in"=w387, "i attribute"=w383, "error in (no error)"=w386) -> ("i ref out"=w388:refnum<vi>, "error out"=w385:errorcluster)  [unwired: 15 in]
                }
                frame True {
                }
              }
            }
            frame Error {
              n110 = call "CoreLib.set data type mismatch.vi"("error in (no error)"=w394, "error source"=w392) -> ("error out"=w393:errorcluster)  [unwired: 17 in]
            }
          }
          n111 = call "MM9.get i attribute.vi"("i ref in"=w360, "error in (no error)"=w359) -> ("i ref out"=w355:refnum<vi>, "i attribute"=w358:T5, "error out"=w356:errorcluster)  [unwired: 15 in]
          n112 = Unbundle By Name(w358) -> ("MMStatus"=w357:T2)
          n113 = call "MM9.SetStatus.vi"("i ref in"=w355, "MMStatusSuccess"=MM9.status."abort_requested" ("MMStatus"), "MMStatusFail"=w357, "ms timeout (10000)"=w351, "error in (no error)"=w356) -> ("i ref out"=w354:refnum<vi>, "error out"=w353:errorcluster)  [unwired: 11 in, 2 out]
          n114 = case shown="True" FALSE ("Case Constant\n(See Context Help)") {
            tunnel: [w397 w402] -> w364
            tunnel: [w396 w401] -> w363
            tunnel: w348 -> [_ w400]
            tunnel: w354 -> [w397 w399]
            tunnel: w353 -> [w396 w398]
            frame False {
            }
            frame True {
              n115 = call "BaseProcess.set event status.vi"("i ref in"=w399, "EventStatus"=w400, "error in (no error)"=w398) -> ("i ref out"=w402:refnum<vi>, "error out"=w401:errorcluster)  [unwired: 14 in, 1 out]
            }
          }
          n116 = case shown="Error" w363 {
            selector: w363 -> [_ w405]
            tunnel: [_ w404] -> w367
            frame No Error {
            }
            frame Error {
              n117 = Unbundle By Name(w405) -> ("source"=w403:string)
              n118 = call-poly "CoreLib.data 2 byte array.vi"("string"=w403) -> ("byteArray out"=w404:T1)  [unwired: 18 in]
            }
          }
          n119 = Unbundle By Name(w363) -> ("code"=w366:i32)
          n120 = Bundle By Name(cluster=w347, "Data"=w367, "Error #"=w366) -> (w365:T3)
        }
        frame "stop" {
          # "\"STOPPROCESS\""
          n121 = Unbundle By Name(w407) -> ("Data"=w406:T1)
          n122 = call-poly "CoreLib.byte array 2 data.vi"("byteArray"=w406) -> ("string"=w409:string, "error out"=w410:errorcluster)  [unwired: 16 in, 1 out]
          n123 = case shown="No Error" w410 {
            tunnel: w428 -> [w434 w450]
            tunnel: w427 -> [w431 w453]
            tunnel: [w438 _] -> _
            tunnel: [w436 w450] -> w420
            tunnel: [w435 w452] -> w419
            tunnel: w412 -> [w429 w454]
            tunnel: [w429 w454] -> w411
            tunnel: w409 -> [w430 _]
            tunnel: w408 -> [_ w451]
            frame No Error {
              n124 = call "MM9.set GUI ID.vi"("i ref in"=w434, "GUIDString"=w430, "ms timeout (10000)"=w429, "error in (no error)"=w431) -> ("i ref out"=w432:refnum<vi>, "error out"=w433:errorcluster)  [unwired: 13 in, 1 out]
              n125 = call "MM9.get data to modify.vi"("i ref in"=w432, "ms timeout (10000)"=w429, "error in (no error)"=w433) -> ("i ref out"=w440:refnum<vi>, "i attribute"=w437:T5, "timed out"=w438:bool, "error out"=w439:errorcluster)  [unwired: 13 in]
              n126 = case "timed out?" shown="False" w438 {
                tunnel: w440 -> [w446 w449]
                tunnel: [w447 w449] -> w436
                tunnel: w439 -> [w445 w448]
                tunnel: [w444 w448] -> w435
                tunnel: w437 -> [w443 _]
                frame False {
                  n127 = Bundle By Name(cluster=w443, "StopRequest"=TRUE ("BreakRequest")) -> (w442:T5)
                  n128 = call "MM9.set modified data.vi"("i ref in"=w446, "i attribute"=w442, "error in (no error)"=w445) -> ("i ref out"=w447:refnum<vi>, "error out"=w444:errorcluster)  [unwired: 15 in]
                }
                frame True {
                }
              }
            }
            frame Error {
              n129 = call "CoreLib.set data type mismatch.vi"("error in (no error)"=w453, "error source"=w451) -> ("error out"=w452:errorcluster)  [unwired: 17 in]
            }
          }
          n130 = call "MM9.get i attribute.vi"("i ref in"=w420, "error in (no error)"=w419) -> ("i ref out"=w415:refnum<vi>, "i attribute"=w418:T5, "error out"=w416:errorcluster)  [unwired: 15 in]
          n131 = Unbundle By Name(w418) -> ("MMStatus"=w417:T2)
          n132 = call "MM9.SetStatus.vi"("i ref in"=w415, "MMStatusSuccess"=MM9.status."stop_requested" ("MMStatus"), "MMStatusFail"=w417, "ms timeout (10000)"=w411, "error in (no error)"=w416) -> ("i ref out"=w414:refnum<vi>, "error out"=w413:errorcluster)  [unwired: 11 in, 2 out]
          n133 = call "BaseProcess.set event status.vi"("i ref in"=w414, "EventStatus"=w408, "error in (no error)"=w413) -> ("i ref out"=w423:refnum<vi>, "error out"=w422:errorcluster)  [unwired: 14 in, 1 out]
          n134 = case shown="Error" w422 {
            selector: w422 -> [_ w457]
            tunnel: [_ w456] -> w426
            frame No Error {
            }
            frame Error {
              n135 = Unbundle By Name(w457) -> ("source"=w455:string)
              n136 = call-poly "CoreLib.data 2 byte array.vi"("string"=w455) -> ("byteArray out"=w456:T1)  [unwired: 18 in]
            }
          }
          n137 = Unbundle By Name(w422) -> ("code"=w425:i32)
          n138 = Bundle By Name(cluster=w407, "Data"=w426, "Error #"=w425) -> (w424:T3)
        }
        frame "quit" {
          n139 = Unbundle By Name(w459) -> ("Data"=w458:T1)
          n140 = call-poly "CoreLib.byte array 2 data.vi"("byteArray"=w458) -> ("string"=w462:string, "error out"=w461:errorcluster)  [unwired: 16 in, 1 out]
          n141 = case shown="No Error" w461 {
            tunnel: [w488 w496] -> w469
            tunnel: [w487 w494] -> w468
            tunnel: w465 -> [w485 w496]
            tunnel: w464 -> [w483 w495]
            tunnel: w463 -> [w482 _]
            tunnel: w462 -> [_ _]
            tunnel: w460 -> [_ w493]
            tunnel: [w480 _] -> _
            frame No Error {
              n142 = call "MM9.set GUI ID.vi"("i ref in"=w485, "GUIDString"="N/A", "ms timeout (10000)"=w482, "error in (no error)"=w483) -> ("i ref out"=w486:refnum<vi>, "timed out"=w480:bool, "error out"=w484:errorcluster)  [unwired: 13 in]
              n143 = call "MM9.get i attribute.vi"("i ref in"=w486, "error in (no error)"=w484) -> ("i ref out"=w492:refnum<vi>, "i attribute"=w490:T5, "error out"=w491:errorcluster)  [unwired: 15 in]
              n144 = Unbundle By Name(w490) -> ("UsedObjs"=w489:string[])
              n145 = call "MM9.UnloadObjs.vi"("i ref in"=w492, "ObjsToUnload"=w489, "error in (no error)"=w491) -> ("i ref out"=w488:refnum<vi>, "error out"=w487:errorcluster)  [unwired: 15 in]
            }
            frame Error {
              n146 = call "CoreLib.set data type mismatch.vi"("error in (no error)"=w495, "error source"=w493) -> ("error out"=w494:errorcluster)  [unwired: 17 in]
            }
          }
          n147 = call "MM9.get i attribute.vi"("i ref in"=w469, "error in (no error)"=w468) -> ("i ref out"=w470:refnum<vi>, "i attribute"=w473:T5, "error out"=w471:errorcluster)  [unwired: 15 in]
          n148 = Unbundle By Name(w473) -> ("MMStatus"=w472:T2)
          n149 = call "MM9.SetStatus.vi"("i ref in"=w470, "MMStatusSuccess"=MM9.status."NOTConnected" ("MMStatus"), "MMStatusFail"=w472, "ms timeout (10000)"=w463, "error in (no error)"=w471) -> ("i ref out"=w467:refnum<vi>, "error out"=w466:errorcluster)  [unwired: 11 in, 2 out]
          n150 = call "BaseProcess.set event status.vi"("i ref in"=w467, "EventStatus"=w460, "error in (no error)"=w466) -> ("i ref out"=w479:refnum<vi>, "error out"=w478:errorcluster)  [unwired: 14 in, 1 out]
          n151 = case shown="No Error" w478 {
            selector: w478 -> [_ w499]
            tunnel: [_ w498] -> w476
            frame No Error {
            }
            frame Error {
              n152 = Unbundle By Name(w499) -> ("source"=w497:string)
              n153 = call-poly "CoreLib.data 2 byte array.vi"("string"=w497) -> ("byteArray out"=w498:T1)  [unwired: 18 in]
            }
          }
          n154 = Unbundle By Name(w478) -> ("code"=w475:i32)
          n155 = Bundle By Name(cluster=w459, "Data"=w476, "Error #"=w475) -> (w477:T3)
        }
        frame "PING" {
          n156 = Unbundle By Name(w501) -> ("Data"=w500:T1)
          n157 = call-poly "CoreLib.byte array 2 data.vi"("byteArray"=w500) -> ("string"=w505:string, "error out"=w506:errorcluster)  [unwired: 16 in, 1 out]
          n158 = case shown="No Error" w506 {
            tunnel: w510 -> [w528 w532]
            tunnel: [w527 w532] -> w509
            tunnel: [w526 w530] -> w508
            tunnel: w507 -> [w525 w531]
            tunnel: w505 -> [w524 _]
            tunnel: w504 -> [w523 w533]
            tunnel: [w523 w533] -> w503
            tunnel: w502 -> [_ w529]
            frame No Error {
              n159 = call "MM9.set GUI ID.vi"("i ref in"=w528, "GUIDString"=w524, "ms timeout (10000)"=w523, "error in (no error)"=w525) -> ("i ref out"=w527:refnum<vi>, "error out"=w526:errorcluster)  [unwired: 13 in, 1 out]
            }
            frame Error {
              n160 = call "CoreLib.set data type mismatch.vi"("error in (no error)"=w531, "error source"=w529) -> ("error out"=w530:errorcluster)  [unwired: 17 in]
            }
          }
          n161 = call "MM9.get i attribute.vi"("i ref in"=w509, "error in (no error)"=w508) -> ("i ref out"=w513:refnum<vi>, "i attribute"=w516:T5, "error out"=w514:errorcluster)  [unwired: 15 in]
          n162 = Unbundle By Name(w516) -> ("MMStatus"=w515:T2)
          n163 = call "MM9.SetStatus.vi"("i ref in"=w513, "MMStatusSuccess"=MM9.status."Connected" ("MMStatus"), "MMStatusFail"=w515, "ms timeout (10000)"=w503, "error in (no error)"=w514) -> ("i ref out"=w512:refnum<vi>, "error out"=w511:errorcluster)  [unwired: 11 in, 2 out]
          n164 = call "BaseProcess.set event status.vi"("i ref in"=w512, "EventStatus"=w502, "error in (no error)"=w511) -> ("i ref out"=w522:refnum<vi>, "error out"=w521:errorcluster)  [unwired: 14 in, 1 out]
          n165 = case shown="Error" w521 {
            selector: w521 -> [_ w536]
            tunnel: [_ w535] -> w519
            frame No Error {
            }
            frame Error {
              n166 = Unbundle By Name(w536) -> ("source"=w534:string)
              n167 = call-poly "CoreLib.data 2 byte array.vi"("string"=w534) -> ("byteArray out"=w535:T1)  [unwired: 18 in]
            }
          }
          n168 = Unbundle By Name(w521) -> ("code"=w518:i32)
          n169 = Bundle By Name(cluster=w501, "Data"=w519, "Error #"=w518) -> (w520:T3)
        }
      }
    }
    frame Error {
    }
  }
  "answer cluster" <- w9
  "i ref out" <- w7
  "error out" <- w6
